vi "Execution.vi"() -> ()   [LabVIEW 2015]
panel:
  in  "Exec Counter":u32
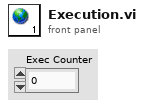
[diagram p1: front panel]
diagram:
